vi "create.request.vi"(8 "error in":errorcluster, 9 "Assets":string[](array[string]), 10 "Start Time":timestamp format="%<%x %.3X>T", 11 "Title":string) -> (0 "error out":errorcluster, 1 "Request":string)   [LabVIEW 2020, in "Run.lvclass"]
uses:
  Run.lvclass
  <vilib>/LabVIEW Open Source Project/Epoch Date & Time/epoch.UNIX/Epoch.UNIX.lvclass
  C:/Program Files/National Instruments/LabVIEW 2026/vi.lib/LabVIEW Open Source Project/Epoch Date & Time/epoch/Epoch.lvclass
  <vilib>/JDP Science/JSONtext/LVClass Serializer/JSONtext LVClass Serializer.lvclass
  2fbe8fca-b16e-45d9-9acc-ed174a081b12.vi
  21ec94b3-9936-4974-8d50-7fe96fbbf006.vi
  f841ec19-bfb9-4846-abda-e87ddc9cbd9d.vi
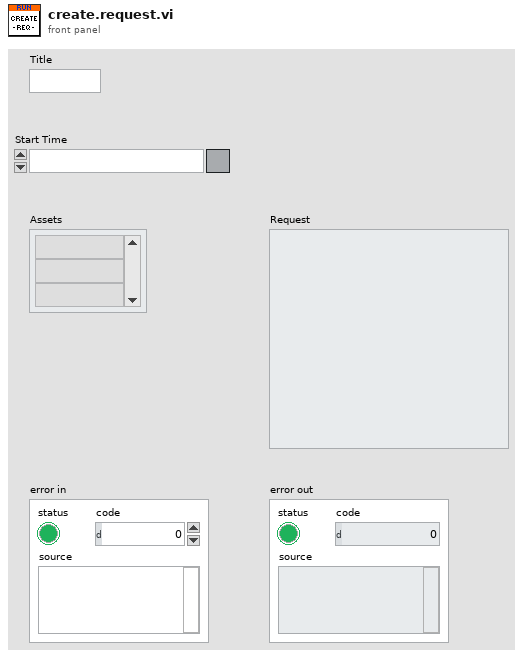
[diagram p1: front panel]
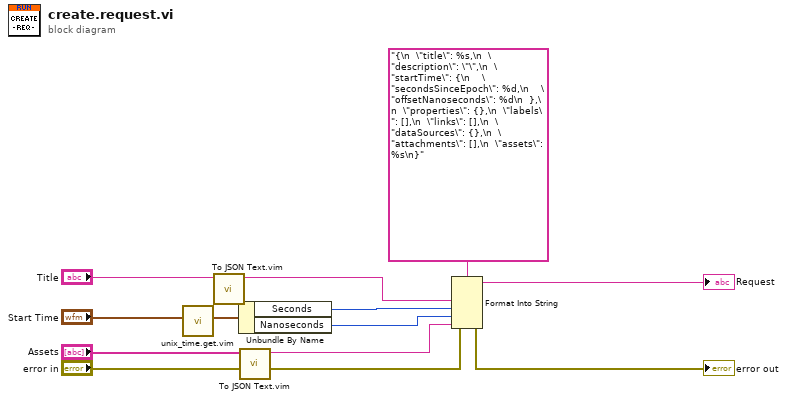
[diagram p0: block diagram]
diagram:
  n1 = call "unix_time.get.vim"("Time Stamp (empty: now) [single or array]"="Start Time") -> ("UNIX Timestamp"=w7:cluster{"Seconds":i64, "Nanoseconds":i64})  [unwired: 10 in]
  n2 = call "To JSON Text.vim"("Anything"="Title") -> ("<JSON>"=w1:string)  [unwired: 9 in, 1 out]
  n3 = Unbundle By Name(w7) -> ("Seconds"=w4:i64, "Nanoseconds"=w5:i64)
  n4 = call "To JSON Text.vim"("error in (no error)"="error in", "Anything"="Assets") -> ("error out"=w3:errorcluster, "<JSON>"=w2:string)  [unwired: 8 in]
  n5 = Format Into String(format string="{\n  \"title\": %s,\n  \"description\": \"\",\n  \"startTime\": {\n    \"secondsSinceEpoch\": %d,\n    \"offsetNanoseconds\": %d\n  },\n  \"properties\": {},\n  \"labels\": [],\n  \"links\": [],\n  \"dataSources\": {},\n  \"attachments\": [],\n  \"assets\": %s\n}", error in=w3, w1, w4, w5, w2) -> (resulting string=→"Request":string, error out=→"error out":errorcluster)  [unwired: 1 in]
